vi "RshTest.vi"() -> ()   [LabVIEW 2017]
uses:
  <vilib>/Utility/file.llb/Read Delimited Spreadsheet (DBL).vi
panel:
  out "appended array":dbl[](array[numeric])
  in  "base path 2":path
  out "Rsh curve over time":cluster{"array":dbl[], "array":dbl[]}(graph)
  out "output Rsh":dbl[][](array[numeric])
  out "Last Rsh (Ohm)":dbl
  in  "number":u16
  out "Rsh":dbl
  in  "file path Rsh":path=path "C:/Users/Jonathan/Documents/UHasselt/Masterproef/LabVEIW/data/24-05-19_11h55/Module1/0.csv"
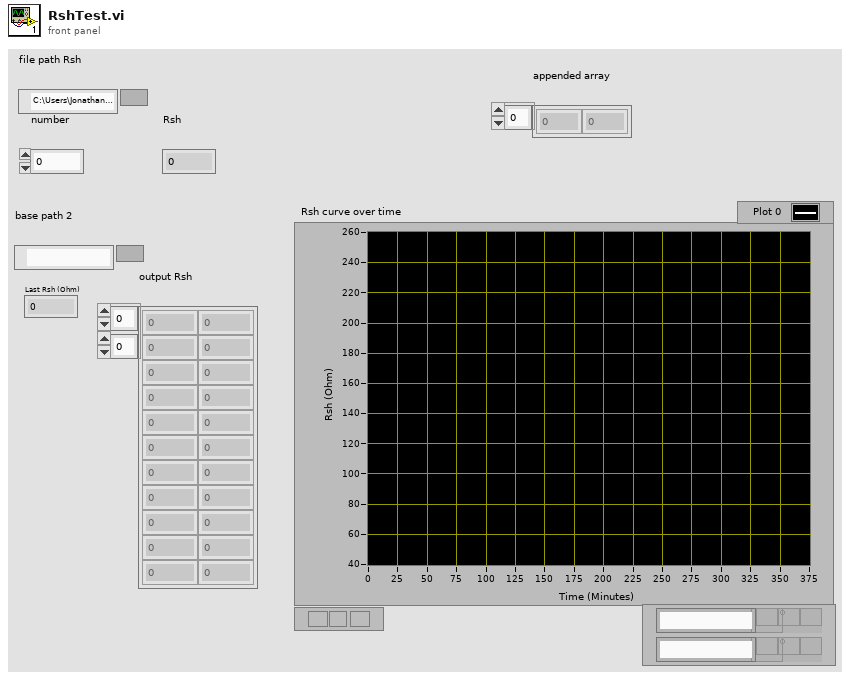
[diagram p1: front panel]
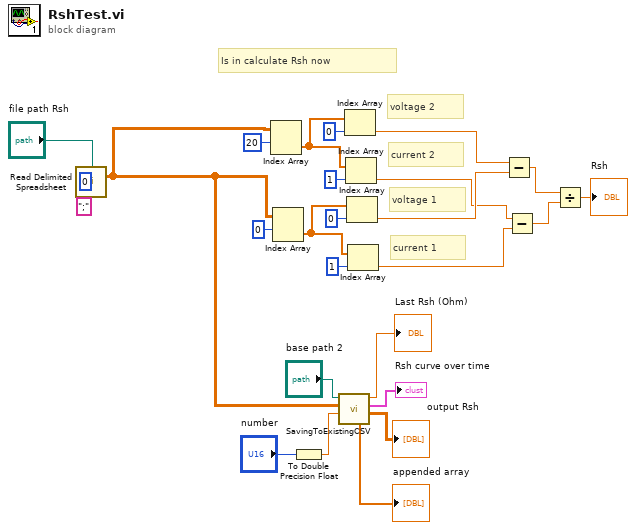
[diagram p0: block diagram]
diagram:
  # "Is in calculate Rsh now"
  # "current 1"
  # "voltage 1"
  # "current 2"
  # "voltage 2"
  n1 = call-poly <vilib>:"Read Delimited Spreadsheet.vi"("file path (dialog if empty)"="file path Rsh", "start of read offset (chars.:0)"=0, "delimiter (\\t)"=";" ("delimiter (\\t)")) -> ("all rows"=w6:dbl[][])  [unwired: 7 in, 5 out]
  n2 = Index Array(array=w6, index (row)=20) -> (element=w19:dbl[])  [unwired: 1 in]
  n3 = Index Array(array=w6, index (row)=0) -> (element=w16:dbl[])  [unwired: 1 in]
  n4 = To Double Precision Float(number="number") -> (double precision float=w5:dbl)
  n5 = call "SavingToExistingCSV.vi"("Numeric"=w5, "all rows"=w6, "base path in"="base path 2") -> ("output array"=→"output Rsh":dbl[][], "XY Graph 4"=→"Rsh curve over time":cluster{"array":dbl[], "array":dbl[]}, "Last Rsh (Ohm)"=→"Last Rsh (Ohm)":dbl, "appended array"=→"appended array":dbl[])  [unwired: 5 in]
  n6 = Index Array(array=w19, index=0) -> (element=w13:dbl)
  n7 = Index Array(array=w19, index=1) -> (element=w11:dbl)
  n8 = Index Array(array=w16, index=0) -> (element=w12:dbl)
  n9 = Index Array(array=w16, index=1) -> (element=w10:dbl)
  n10 = Subtract(x=w13, y=w12) -> (x-y=w15:dbl)
  n11 = Subtract(x=w11, y=w10) -> (x-y=w14:dbl)
  n12 = Divide(x=w15, y=w14) -> (x/y=→"Rsh":dbl)
